vi "FindTagMatches.vi"(10 "All Tags":string[](array[string]), 11 "NameToFind":string) -> (1 "Not Found":string[](array[string]), 2 "Found":string[](array[string]), 3 "ResultString":string)   [LabVIEW 2013, in "FindName Task_Manager.lvlib"]
doc: "Find all tags that match name"
uses:
  FindName Task_Manager.lvlib
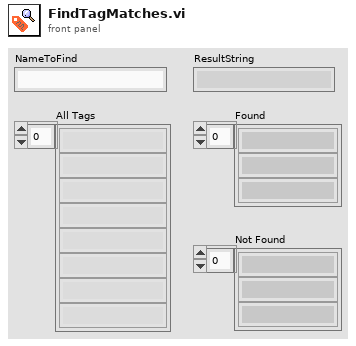
[diagram p1: front panel]
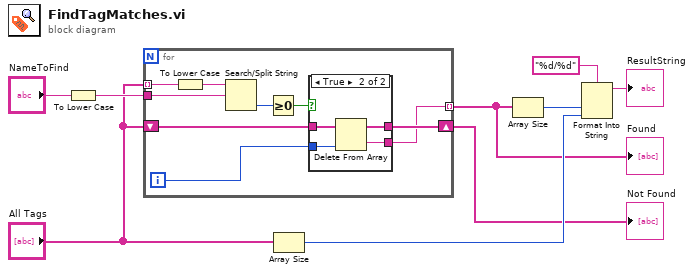
[diagram p0: block diagram]
diagram:
  n1 = To Lower Case(string="NameToFind") -> (all lower case string=w4:string)
  n2 = for {
    tunnel: w4 -> [w15]
    tunnel: "All Tags" -> [w16] mode=indexing
    shift-right: [w13] -> w1
    shift-left: "All Tags" -> [w14]
    tunnel: [w11] -> w2 mode=indexing
    i -> [w10]
    n3 = To Lower Case(string=w16) -> (all lower case string=w17:string)
    n4 = Search/Split String(string=w17, search string/char (-)=w15) -> (offset of match=w18:i32)  [unwired: 1 in, 2 out]
    n5 = Greater Or Equal To 0?(x=w18) -> (x >= 0?=w12:bool)
    n6 = case shown="True" w12 {
      tunnel: w14 -> [w19 w23]
      tunnel: [w19 w22] -> w13
      tunnel: w10 -> [_ w21]
      tunnel: [_ w20] -> w11
      frame False {
      }
      frame True {
        n7 = Delete From Array(array=w23, index=w21) -> (deleted portion=w20:string, array with subset deleted=w22:string[])  [unwired: 1 in]
      }
    }
  }
  "Found" <- w2
  "Not Found" <- w1
  n8 = Array Size(array="All Tags") -> (size(s)=w7:i32)
  n9 = Array Size(array=w2) -> (size(s)=w8:i32)
  n10 = Format Into String(format string="%d/%d", w8, w7) -> (resulting string=→"ResultString":string)  [unwired: 2 in, 1 out]
